vi "Get Channel Properties.vi"(8 "error in":errorcluster, 10 "Channel Details":T1, 11 "TDMS in":refnum<class "TDMS.lvclass">) -> (0 "error out":errorcluster, 2 "Channel Details out":T1, 3 "TDMS out":refnum<class "TDMS.lvclass">)   [LabVIEW 2019, in "TDMS.lvlib" / "TDMS.lvclass"]
uses:
  TDMS.lvclass
  Custom Controls/Group Properties.ctl
  Custom Controls/Channel Properties.ctl
  TDMS.lvclass/TDMS.ctl
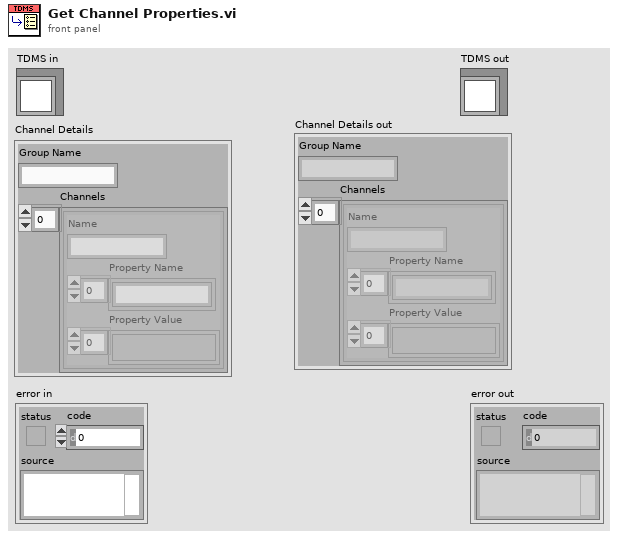
[diagram p1: front panel]
types:
  T1 = typedef "TDMS.lvlib/TDMS.lvclass/Group Properties.ctl" = cluster{"Group Name":string, "Channels":T2[]}
  T2 = typedef "TDMS.lvlib/TDMS.lvclass/Channel Properties.ctl" = cluster{"Name":string, "Property Name":string[], "Property Value":variant[]}
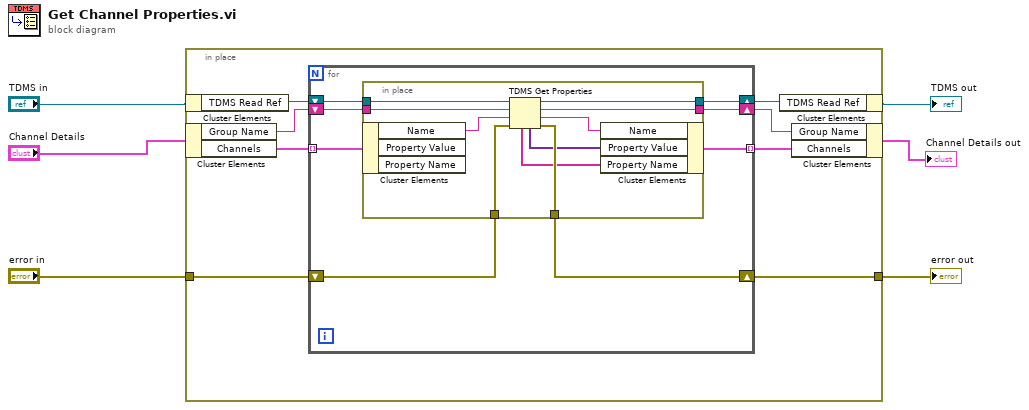
[diagram p0: block diagram]
diagram:
  n1 = in-place {
    in-place-border: [w12] -> w3
    in-place-border: "error in" -> [w11]
    n2 = in-place-cluster #1("TDMS in") -> ("TDMS Read Ref"=w14:refnum<k34>)
    n3 = in-place-cluster #2("Channel Details") -> ("Group Name"=w10:string, "Channels"=w8:T2[])
    n4 = for {
      shift-right: [w21] -> w13
      shift-left: w14 -> [w22]
      shift-right: [w20] -> w12
      shift-left: w11 -> [w19]
      shift-right: [w17] -> w9
      shift-left: w10 -> [w18]
      tunnel: w8 -> [w16] mode=indexing
      tunnel: [w15] -> w7 mode=indexing
      n5 = in-place {
        in-place-border: w22 -> [w32]
        in-place-border: [w31] -> w21
        in-place-border: [w30] -> w20
        in-place-border: w19 -> [w29]
        in-place-border: w18 -> [w28]
        in-place-border: [w27] -> w17
        n6 = in-place-cluster #3(w16) -> ("Name"=w26:string)  [unwired: 2 out]
        n7 = TDMS Get Properties(8:w29, 9:w26, 10:w28, 11:w32) -> (0:w30:errorcluster, 1:w25:string, 2:w27:string, 3:w31:refnum<k34>, 4:w24:variant[], 6:w23:string[])  [unwired: 2 in]
        n8 = in-place-cluster #3("Name"=w25, "Property Value"=w24, "Property Name"=w23) -> (w15:T2)
      }
    }
    n9 = in-place-cluster #1("TDMS Read Ref"=w13) -> (→"TDMS out":refnum<class "TDMS.lvclass">)
    n10 = in-place-cluster #2("Group Name"=w9, "Channels"=w7) -> (→"Channel Details out":T1)
  }
  "error out" <- w3
